vi "get inverter SN.vi"(8 "error in":errorcluster, 10 "File counter":i32, 11 "Config in":refnum<class "Config.lvclass">) -> (0 "error out":errorcluster, 1 "File namd":string[](array[string]), 2 "BaseFN":string[](array[string])=["DUT1", "DUT2", "DUT3", "DUT4"], 3 "Config out":refnum<class "Config.lvclass">)   [LabVIEW 2019, in "Log_Engine.lvclass"]
uses:
  Log_Engine.lvclass
  Config/Config.lvclass
  Common/DataTypes/Inverter LUT v2--cluster.ctl
  Common/DataTypes/Inverter database record v2--cluster.ctl
  Common/DataTypes/inverter info v2--cluster.ctl
  Common/DataTypes/inverter gain range--cluster.ctl
  Common/DataTypes/inverter offset range--cluster.ctl
  Config/Config.lvclass/Config.ctl
  Config/Accessors/Get Main Settings.vi
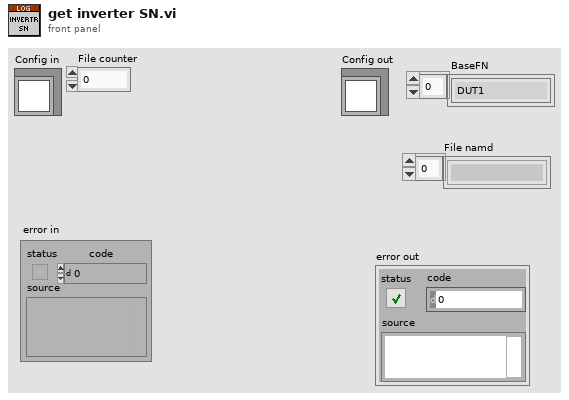
[diagram p1: front panel]
types:
  T1 = typedef "Inverter LUT v2--cluster.ctl" = cluster{"Inverter Records":T2[]}
  T2 = typedef "Inverter database record v2--cluster.ctl" = cluster{"name":string, "last updated":timestamp, "type":string, "inverter Info":T3, "gain range":T4, "offset range":T5, "gain actual":dbl, "offset actual":dbl, "power level":dbl, "minimum current":dbl, "resistance single phase":dbl, "resistance 3 phase":dbl, "set flag":u16}
  T3 = typedef "inverter info v2--cluster.ctl" = cluster{"manufacturer":string, "model":string, "product":string, "serial":string, "power class":string, "year manf":string}
  T4 = typedef "inverter gain range--cluster.ctl" = cluster{"gain max":dbl, "gain min":dbl, "gain increment":dbl}
  T5 = typedef "inverter offset range--cluster.ctl" = cluster{"offset max":dbl, "offset min":dbl, "offset increment":dbl}
  T6 = typedef "Main.lvclass/Settings--cluster.ctl" = cluster{"Simulation":bool, "Signal scaling":T7[], "ESR scaling":T8[], "num readings to average":i32[], "ESR alarm threshhold (%)":i32[], "UseDummyVrms":bool, "Dummy Vrms":dbl, "Inverter Database File":path, "default Inverter (name)":string[]}
  T7 = typedef "Main.lvclass/Gain control.ctl" = cluster{"Iin ripple gain":dbl, "Iout ripple gain":dbl, "Iout 60Hz gain ":dbl, "Vout 60Hz gain ":dbl, "Iin ripple offest":dbl, "Iout ripple offset":dbl, "Iout 60Hz offset":dbl, "Vout 60Hz offset":dbl}
  T8 = typedef "Main.lvclass/ESR scaling--cluster.ctl" = cluster{"Gain":dbl, "Offset":dbl}
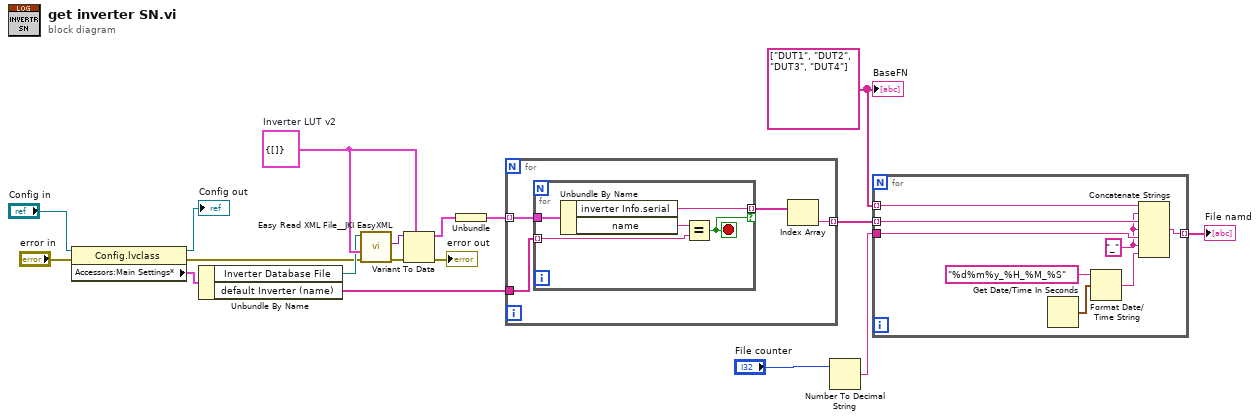
[diagram p0: block diagram]
diagram:
  w9 = string[] ["DUT1", "DUT2", "DUT3", "DUT4"] ("TDMS BaseFN")
  w14 = T1 {"Inverter Records"=[]}  # Inverter LUT v2
  n1 = property class="Config.lvclass"(reference="Config in", error in="error in") -> (reference out=→"Config out":refnum<class "Config.lvclass">, error out=w2:errorcluster, "Accessors:Main Settings*"=w18:T6)
  n2 = Unbundle By Name(w18) -> ("Inverter Database File"=w13:path, "default Inverter (name)"=w11:string[])
  n3 = call <vilib>:"Easy Read XML File__JKI EasyXML.vi"("error in (no error)"=w2, "LabVIEW Data (Type)"=w14, "XML File Path"=w13) -> ("error out"=w15:errorcluster, "LabVIEW Data"=w16:variant)  [unwired: 6 in, 1 out]
  n4 = Variant To Data(error in=w15, type=w14, Variant=w16) -> (data=w17:T1, error out=→"error out":errorcluster)
  n5 = Unbundle(w17) -> ("Inverter Records"=w12:T2[])
  n6 = for {
    tunnel: w12 -> [w22] mode=indexing
    tunnel: w11 -> [w21]
    tunnel: [w19] -> w7 mode=indexing
    n7 = for {
      tunnel: w22 -> [w27]
      tunnel: w21 -> [w25] mode=indexing
      tunnel: [w24] -> w20 mode=indexing if=w23
      stop <- w23 stop-if-true
      n8 = Unbundle By Name(w27) -> ("inverter Info.serial"=w24:string, "name"=w26:string)
      n9 = Equal?(x=w26, y=w25) -> (x = y?=w23:bool)
    }
    n10 = Index Array(array=w20) -> (element=w19:string)  [unwired: 1 in]
  }
  n11 = Number To Decimal String(number="File counter") -> (decimal integer string=w6:string)  [unwired: 1 in]
  n12 = for {
    tunnel: w9 -> [w31] mode=indexing
    tunnel: w7 -> [w32] mode=indexing
    tunnel: w6 -> [w30]
    tunnel: [w28] -> w5 mode=indexing
    w29 = "_"
    n13 = Get Date/Time In Seconds() -> (seconds since 1Jan1904=w35:timestamp)
    n14 = Format Date/Time String(time format string (%c)="%d%m%y_%H_%M_%S", seconds (now)=w35) -> (date/time string=w33:string)  [unwired: 1 in]
    n15 = Concatenate Strings(w31, w29, w32, w29, w30, w29, w33) -> (w28:string)
  }
  "File namd" <- w5
  "BaseFN" <- w9
